vi "LoopTermperatureMeanStddev.vi"(8 "error in 2":errorcluster) -> (0 "error out 2":errorcluster, 2 "Temperature Error":dbl=200.0 format="%.2f", 3 "Temperature":dbl=200.0 format="%.2f")   [LabVIEW 2010]
uses:
  <vilib>/Analysis/NI_AALBase.lvlib
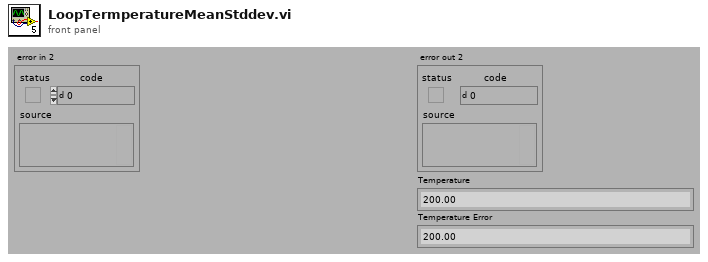
[diagram p1: front panel]
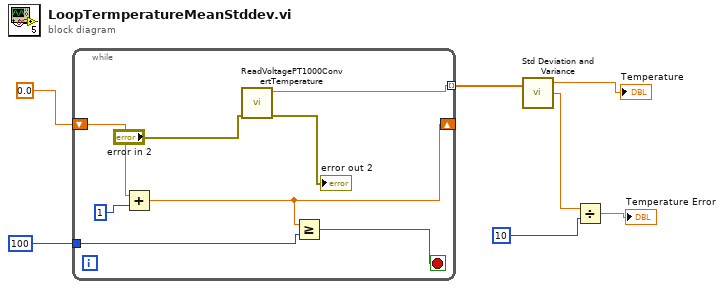
[diagram p0: block diagram]
diagram:
  n1 = while {
    tunnel: 100 -> [w13]
    shift-right: [w12] -> _
    shift-left: 0.0 -> [w14]
    tunnel: [w10] -> w1 mode=indexing
    stop <- w11 stop-if-true
    n2 = Add(x=w14, y=1) -> (x+y=w12:dbl)
    n3 = call "ReadVoltagePT1000ConvertTemperature.vi"("error in 2"="error in 2") -> ("error out 2"=→"error out 2":errorcluster, "Temperature"=w10:dbl)  [unwired: 9 in]
    n4 = Greater Or Equal?(x=w12, y=w13) -> (x >= y?=w11:bool)
  }
  n5 = call <vilib>:"Std Deviation and Variance.vi"("X"=w1) -> ("mean"=→"Temperature":dbl, "standard deviation"=w2:dbl)  [unwired: 1 in, 1 out]
  n6 = Divide(x=w2, y=10) -> (x/y=→"Temperature Error":dbl)
